vi "Message to uService.vi"(0 "Father of all uServices in":refnum<class "Father of all uServices.lvclass">, 5 "uService ID":string, 7 "Message":string, 9 "Data":variant, 11 "error in (no error)":errorcluster, 12 "Locale?":bool) -> (4 "Father of all uServices out":refnum<class "Father of all uServices.lvclass">, 15 "error out":errorcluster)   [LabVIEW 2026, in "TALOS.lvlib" / "Father of all uServices.lvlib" / "Father of all uServices.lvclass"]
doc: "Use this VI to send a message to another uService, using its ID. The target uService has to have a case, inside the Event Handler -> Message case, called as the string passed in Message to this VI. Data is optional.\nBy default, the VI will only send the message to uServices in locale: if Locale? = False, then the VI will try to send the message also to all the uServices with that name running across the network (for now it works only for the uServices instantiated statically at boot, i.e. the ones indicated in AEgIS_Param.ini)."
uses:
  Father of all uServices.lvclass
  C:/LabVIEW Code/TALOS/builds/Actor Framework PPL/Actor Framework.lvlibp/1abvi3w/vi.lib/ActorFramework/Actor/Actor.lvclass
  Guardian/Guardian Messages/Message to uService Msg/Message to uService Msg.lvclass/Message to uService Msg.ctl
  Ancestor/Ancestor/Ancestor.lvclass/Ancestor.ctl
  Support VIs/Generate Error.vi
  FGV/Error Memory/Get Error Description.vi
  Support VIs/Get PC name.vi
  Ancestor/Ancestor/Read ID.vi
  Support VIs/Get Class Name.vi
  <vilib>/Utility/error.llb/Clear Errors.vi
  FGV/Error Memory/Error Memory Core.vi
  <vilib>/AdvancedString/Delimited String to 1D String Array.vi
  <vilib>/AdvancedString/Delimited String to 1D String Array (string).vi
  Support VIs/Circus Root Path.vi
  FGV/Error Memory/Error Crt Lvl checker.vi
  FGV/Error Memory/Error Memory Core.vi/40c8088d-b597-4017-91af-faa98e00292e.vi
  FGV/Error Memory/Error Memory Core.vi/d4a3ab98-063c-4e44-b43d-fbdcfe6c2be2.vi
  builds/Actor Framework PPL/Actor Framework.lvlibp/1abvi3w/vi.lib/ActorFramework/Message Enqueuer/Enqueue.vi
  Support VIs/Global Memory.vi
  <vilib>/Utility/LVClass/Get LV Class Name.vi
  Support VIs/Is in Packed Library.vi
  Support VIs/TALOS Root path.vi
  Support VIs/Read CSV worksheet.vi
  Support VIs/Global Constants.vi
  <vilib>/Utility/error.llb/General Error Handler.vi
  Support VIs/Error Log.vi
  Guardian/Guardian Messages/Message to uService Msg/Message to uService Msg.lvclass
  Ancestor/Ancestor/Ancestor.lvclass
  <vilib>/Comparison/Equal/Equal Functor/Equal Functor.lvclass
  builds/Actor Framework PPL/Actor Framework.lvlibp/1abvi3w/vi.lib/ActorFramework/Actor/Actor.lvclass
  TALOS.lvlib
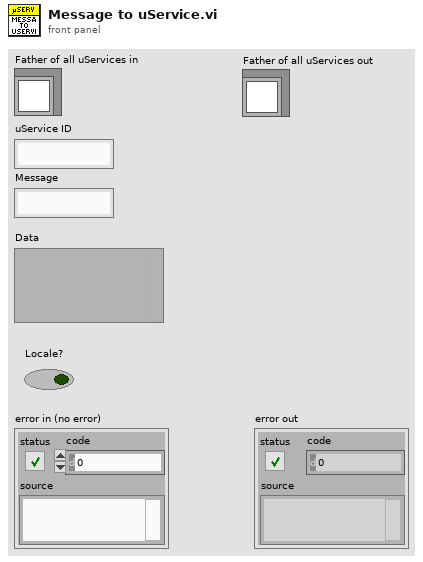
[diagram p1: front panel]
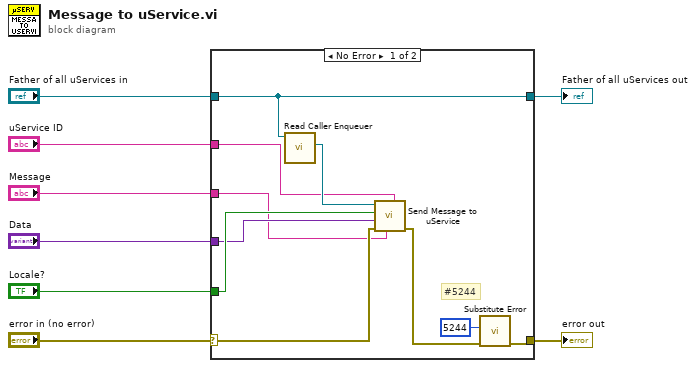
[diagram p0: block diagram]
diagram:
  n1 = case shown="No Error" "error in (no error)" {
    selector: "error in (no error)" -> [w14 w20]
    tunnel: [w10 w20] -> w7
    tunnel: "uService ID" -> [w12 _]
    tunnel: "Message" -> [w13 _]
    tunnel: "Data" -> [w15 _]
    tunnel: "Father of all uServices in" -> [w18 w19]
    tunnel: [w18 w19] -> w2
    tunnel: "Locale?" -> [w16 _]
    frame No Error {
      # "#5244"
      n2 = call "Read Caller Enqueuer.vi"("Actor"=w18) -> ("Caller Enqueuer"=w17:refnum<class "Message Enqueuer.lvclass">)  [unwired: 10 in]
      n3 = call "Send Message to uService.vi"("uService ID"=w12, "Message"=w13, "error in (no error)"=w14, "Data"=w15, "Locale?"=w16, "Message Enqueuer"=w17) -> ("error out"=w9:errorcluster)  [unwired: 4 in, 1 out]
      n4 = call "Substitute Error.vi"("error in (no error)"=w9, "Error Code"=5244) -> ("error out"=w10:errorcluster)  [unwired: 9 in]
    }
    frame Error {
    }
  }
  "error out" <- w7
  "Father of all uServices out" <- w2
